vi "Mercury Temperature monitor 2.vi"() -> ()   [LabVIEW 2014]
uses:
  <vilib>/Utility/file.llb/Write To Spreadsheet File (DBL).vi
panel:
  in  "Data Information":string
  out "Needle valve gearing":dbl
  in  "Needle valve gearing":i8
  in  "Needle valve position":dbl(slide) scale=0.0..100.0
  out "Flow set":bool
  out "He-4 flow":dbl
  in  "K pot heater voltage":dbl
  in  "K pot heater":bool
  out "He-3 pot HTR voltage":dbl
  out "Sorb HTR voltage":dbl
  in  "Sorb heater voltage":dbl
  in  "Sorb heater":bool
  out "Sorb Graph":dbl[][](graph)
  in  "seconds to wait":u32=1
  out "General Graph":dbl[][](graph)
  out "He-3 high":dbl
  out "He-3 low":dbl
  out "K pot":dbl
  out "Sorb":dbl
  in  "stop":bool
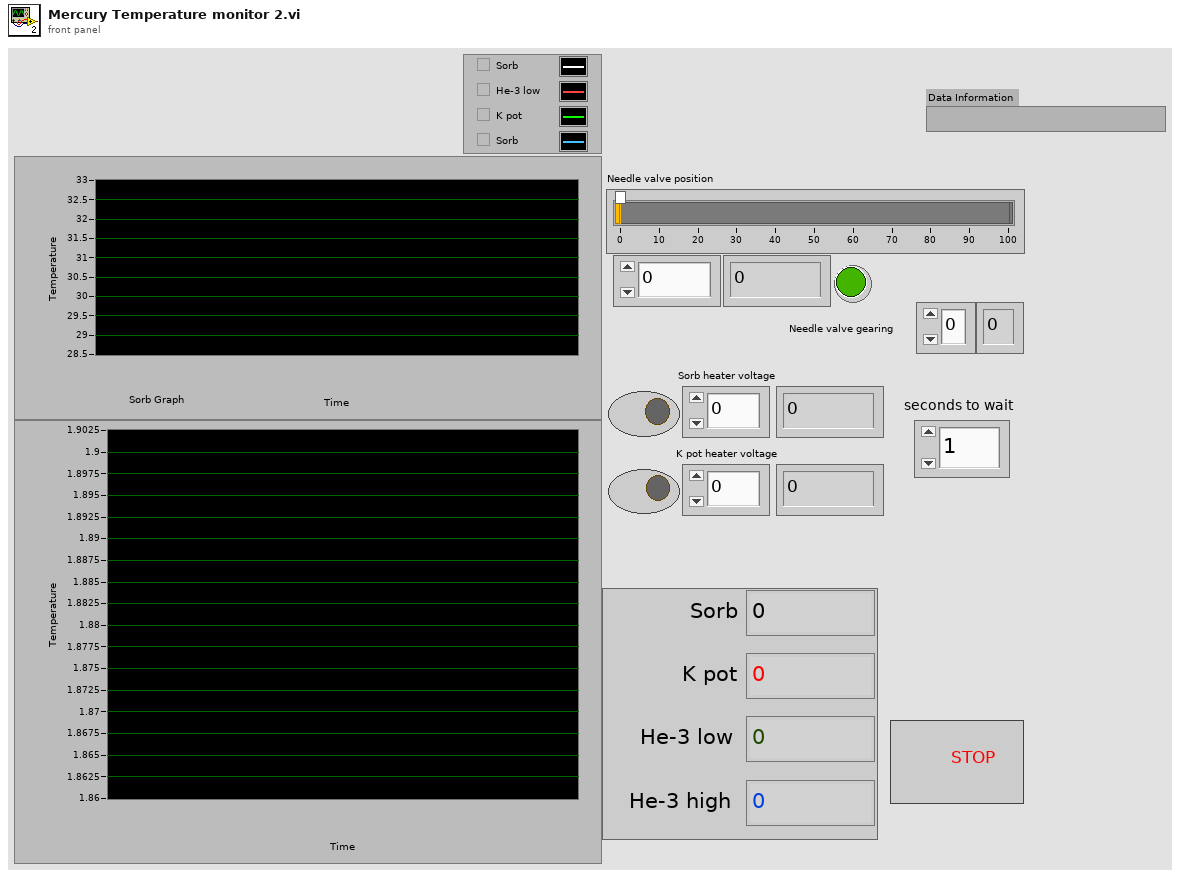
[diagram p1: front panel]
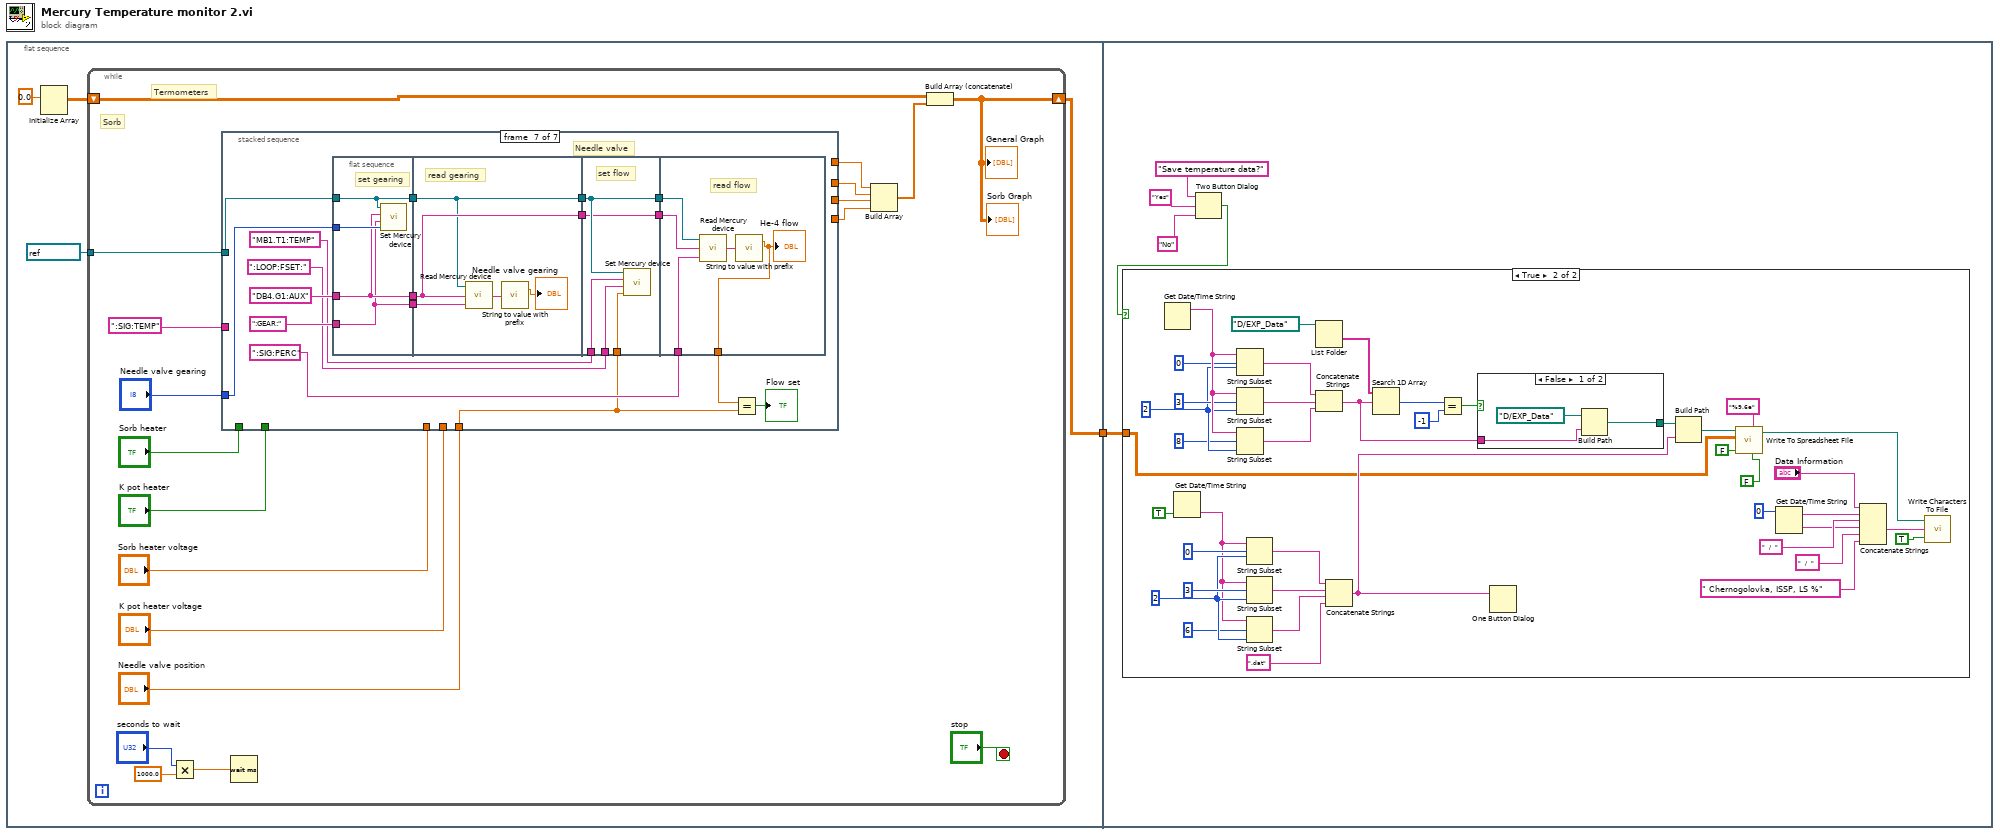
[diagram p0: block diagram]
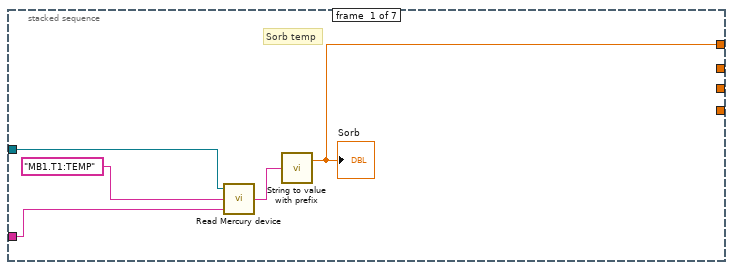
[diagram p2: hidden frame]
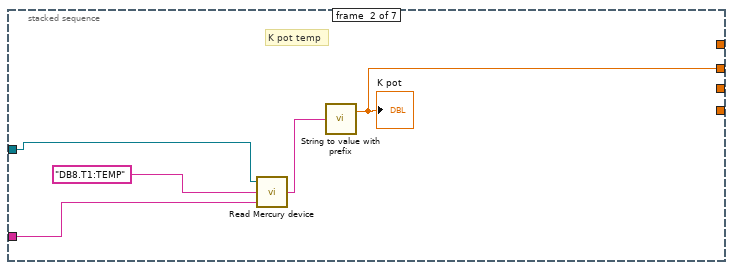
[diagram p3: hidden frame]
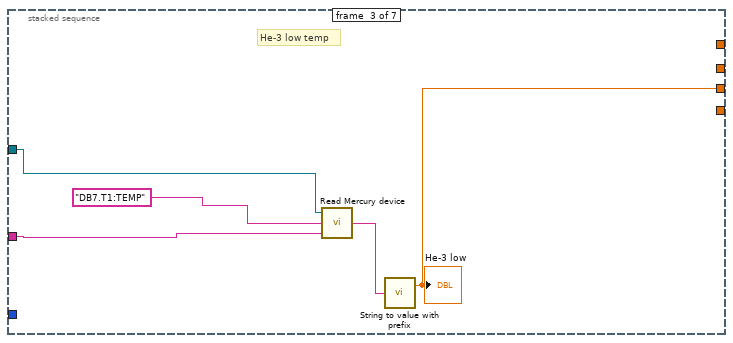
[diagram p4: hidden frame]
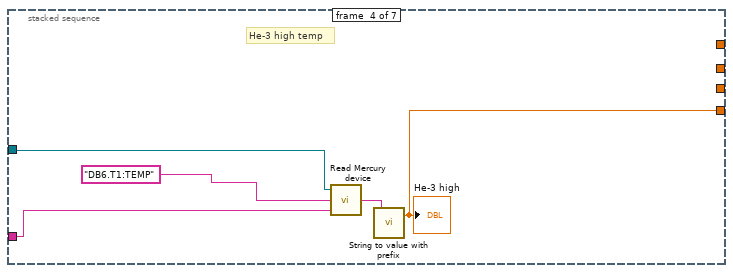
[diagram p5: hidden frame]
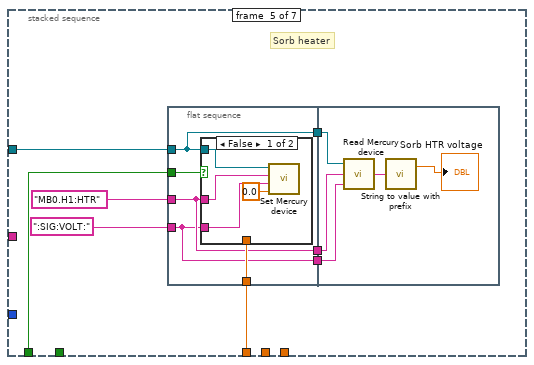
[diagram p6: hidden frame]
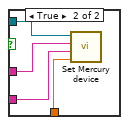
[diagram p7: hidden frame]
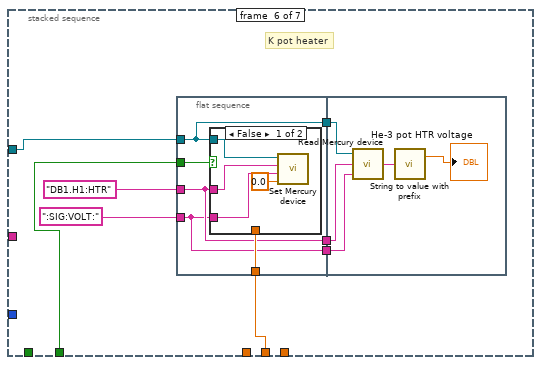
[diagram p8: hidden frame]
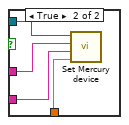
[diagram p9: hidden frame]
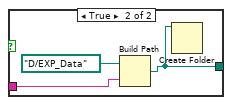
[diagram p11: hidden frame]
diagram:
  n1 = flat-sequence {
    tunnel: [w2] -> w1
    tunnel: w1 -> [w133]
    frame #0 {
      n2 = Initialize Array(0.0 ("element")) -> (w3:dbl[][])  [unwired: 2 in]
      n3 = while {
        shift-right: [w6] -> w2
        shift-left: w3 -> [w7]
        tunnel: refnum<visa-resource-name> "COM4" ("VISA resource name") -> [w23]
        stop <- "stop" stop-if-true
        # "Sorb"
        # "Termometers"
        n4 = Multiply(x="seconds to wait", y=1000.0) -> (x*y=w17:dbl)
        n5 = stacked-sequence {
          tunnel: w23 -> [w29 w33 w39 w43 w48 w73 w112]
          tunnel: ":SIG:TEMP" -> [w28 w34 w38 w42 _ _ _]
          tunnel: [w25 _ _ _ _ _ _] -> w15
          tunnel: [_ w30 _ _ _ _ _] -> w21
          tunnel: [_ _ w35 _ _ _ _] -> w20
          tunnel: [_ _ _ w40 _ _ _] -> w19
          tunnel: "Sorb heater" -> [_ _ _ _ w52 _ _]
          tunnel: "Sorb heater voltage" -> [_ _ _ _ w49 _ _]
          tunnel: "K pot heater" -> [_ _ _ _ _ w72 _]
          tunnel: "K pot heater voltage" -> [_ _ _ _ _ w71 _]
          tunnel: "Needle valve position" -> [_ _ _ _ _ _ w108]
          tunnel: "Needle valve gearing" -> [_ _ _ _ _ _ w105]
          frame #0 {
            # "Sorb temp"
            n6 = call "Read Mercury device.vi"("Additional command"=w28, "Device name"="MB1.T1:TEMP" ("Device Identifier"), "VISA resource name"=w29) -> ("read buffer"=w26:string)
            n7 = call "String to value with prefix.vi"("Incoming string"=w26) -> ("Value"=w25:dbl)  [unwired: 1 out]
            "Sorb" <- w25
          }
          frame #1 {
            # "K pot temp"
            n8 = call "Read Mercury device.vi"("Additional command"=w34, "Device name"="DB8.T1:TEMP" ("Device Identifier"), "VISA resource name"=w33) -> ("read buffer"=w31:string)
            n9 = call "String to value with prefix.vi"("Incoming string"=w31) -> ("Value"=w30:dbl)  [unwired: 1 out]
            "K pot" <- w30
          }
          frame #2 {
            # "He-3 low temp"
            n10 = call "Read Mercury device.vi"("Additional command"=w38, "Device name"="DB7.T1:TEMP" ("Device Identifier"), "VISA resource name"=w39) -> ("read buffer"=w36:string)
            n11 = call "String to value with prefix.vi"("Incoming string"=w36) -> ("Value"=w35:dbl)  [unwired: 1 out]
            "He-3 low" <- w35
          }
          frame #3 {
            # "He-3 high temp"
            n12 = call "Read Mercury device.vi"("Additional command"=w42, "Device name"="DB6.T1:TEMP" ("Device Identifier"), "VISA resource name"=w43) -> ("read buffer"=w41:string)
            n13 = call "String to value with prefix.vi"("Incoming string"=w41) -> ("Value"=w40:dbl)  [unwired: 1 out]
            "He-3 high" <- w40
          }
          frame #4 {
            # "Sorb heater"
            n14 = flat-sequence {
              tunnel: w52 -> [w57]
              tunnel: "MB0.H1:HTR" ("Device Identifier") -> [w54]
              tunnel: ":SIG:VOLT:" ("Device Identifier") -> [w53]
              tunnel: w49 -> [w56]
              tunnel: w48 -> [w55]
              tunnel: [w55] -> w47
              tunnel: [w54] -> w46
              tunnel: [w53] -> w45
              tunnel: w47 -> [w70]
              tunnel: w46 -> [w69]
              tunnel: w45 -> [w68]
              frame #0 {
                n15 = case shown="False" w57 {
                  tunnel: w54 -> [w60 w65]
                  tunnel: w53 -> [w59 w64]
                  tunnel: w56 -> [_ w63]
                  tunnel: w55 -> [w61 w62]
                  frame False {
                    n16 = call "Set Mercury device.vi"("Value"=0.0, "Additional command"=w59, "Device name"=w60, "VISA resource name"=w61) -> ()  [unwired: 1 out]
                  }
                  frame True {
                    n17 = call "Set Mercury device.vi"("Value"=w63, "Additional command"=w64, "Device name"=w65, "VISA resource name"=w62) -> ()  [unwired: 1 out]
                  }
                }
              }
              frame #1 {
                n18 = call "Read Mercury device.vi"("Additional command"=w68, "Device name"=w69, "VISA resource name"=w70) -> ("read buffer"=w67:string)
                n19 = call "String to value with prefix.vi"("Incoming string"=w67) -> ("Value"=→"Sorb HTR voltage":dbl)  [unwired: 1 out]
              }
            }
          }
          frame #5 {
            # "K pot heater"
            n20 = flat-sequence {
              tunnel: w72 -> [w83]
              tunnel: "DB1.H1:HTR" ("Device Identifier") -> [w80]
              tunnel: ":SIG:VOLT:" ("Device Identifier") -> [w79]
              tunnel: w71 -> [w82]
              tunnel: w73 -> [w81]
              tunnel: [w81] -> w78
              tunnel: [w80] -> w77
              tunnel: [w79] -> w76
              tunnel: w78 -> [w96]
              tunnel: w77 -> [w95]
              tunnel: w76 -> [w94]
              frame #0 {
                n21 = case shown="False" w83 {
                  tunnel: w80 -> [w86 w91]
                  tunnel: w79 -> [w85 w90]
                  tunnel: w82 -> [_ w89]
                  tunnel: w81 -> [w87 w88]
                  frame False {
                    n22 = call "Set Mercury device.vi"("Value"=0.0, "Additional command"=w85, "Device name"=w86, "VISA resource name"=w87) -> ()  [unwired: 1 out]
                  }
                  frame True {
                    n23 = call "Set Mercury device.vi"("Value"=w89, "Additional command"=w90, "Device name"=w91, "VISA resource name"=w88) -> ()  [unwired: 1 out]
                  }
                }
              }
              frame #1 {
                n24 = call "Read Mercury device.vi"("Additional command"=w94, "Device name"=w95, "VISA resource name"=w96) -> ("read buffer"=w93:string)
                n25 = call "String to value with prefix.vi"("Incoming string"=w93) -> ("Value"=→"He-3 pot HTR voltage":dbl)  [unwired: 1 out]
              }
            }
          }
          frame #6 {
            # "Needle valve"
            n26 = flat-sequence {
              tunnel: w112 -> [w117]
              tunnel: [w117] -> w104
              tunnel: "DB4.G1:AUX" ("Device Identifier") -> [w115]
              tunnel: ":GEAR:" ("Additional command") -> [w114]
              tunnel: w105 -> [w116]
              tunnel: [w115] -> w100
              tunnel: [w114] -> w97
              tunnel: w104 -> [w119]
              tunnel: [w119] -> w103
              tunnel: w100 -> [w120]
              tunnel: [w120] -> w99
              tunnel: w97 -> [w118]
              tunnel: w108 -> [w127]
              tunnel: [w126] -> w113
              tunnel: w103 -> [w126]
              tunnel: "MB1.T1:TEMP" ("Device Identifier") -> [w125]
              tunnel: ":LOOP:FSET:" ("Device Identifier") -> [w124]
              tunnel: w99 -> [w123]
              tunnel: [w123] -> w98
              tunnel: w113 -> [w132]
              tunnel: ":SIG:PERC" ("Additional command") -> [w130]
              tunnel: [w129] -> w109
              tunnel: w98 -> [w128]
              frame #0 {
                # "set gearing"
                n27 = call "Set Mercury device.vi"("Value"=w116, "Additional command"=w114, "Device name"=w115, "VISA resource name"=w117) -> ()  [unwired: 1 out]
              }
              frame #1 {
                # "read gearing"
                n28 = call "Read Mercury device.vi"("Additional command"=w118, "Device name"=w120, "VISA resource name"=w119) -> ("read buffer"=w122:string)
                n29 = call "String to value with prefix.vi"("Incoming string"=w122) -> ("Value"=→"Needle valve gearing":dbl)  [unwired: 1 out]
              }
              frame #2 {
                # "set flow"
                n30 = call "Set Mercury device.vi"("Value"=w127, "Additional command"=w124, "Device name"=w125, "VISA resource name"=w126) -> ()  [unwired: 1 out]
              }
              frame #3 {
                # "read flow"
                n31 = call "Read Mercury device.vi"("Additional command"=w130, "Device name"=w128, "VISA resource name"=w132) -> ("read buffer"=w131:string)
                n32 = call "String to value with prefix.vi"("Incoming string"=w131) -> ("Value"=w129:dbl)  [unwired: 1 out]
                "He-4 flow" <- w129
              }
            }
            n33 = Equal?(x=w109, y=w108) -> (x = y?=→"Flow set":bool)
          }
        }
        n34 = Wait (ms)(milliseconds to wait=w17) -> ()  [unwired: 1 out]
        n35 = Build Array(w15, w21, w20, w19) -> (w18:dbl[])
        n36 = Build Array (concatenate)(w7, w18) -> (w6:dbl[][])
        "General Graph" <- w6
        "Sorb Graph" <- w6
      }
    }
    frame #1 {
      n37 = Two Button Dialog(message="Save temperature data?", 1:"No" ("F button name (\"Cancel\")"), 2:"Yes" ("T button name (\"OK\")")) -> (T button?=w134:bool)
      n38 = case shown="True" w134 {
        tunnel: w133 -> [_ w139]
        frame False {
        }
        frame True {
          w162 = 2 ("length")
          w174 = 2 ("length")
          n39 = Get Date/Time String() -> (date string=w178:string)  [unwired: 3 in, 1 out]
          n40 = Get Date/Time String(want seconds? (F)=TRUE) -> (time string=w138:string)  [unwired: 2 in, 1 out]
          n41 = String Subset(string=w178, offset (0)=0, length (rest)=w174) -> (substring=w176:string)
          n42 = String Subset(string=w178, offset (0)=3, length (rest)=w174) -> (substring=w172:string)
          n43 = String Subset(string=w178, offset (0)=8, length (rest)=w174) -> (substring=w171:string)
          n44 = String Subset(string=w138, offset (0)=0, length (rest)=w162) -> (substring=w164:string)
          n45 = String Subset(string=w138, offset (0)=3, length (rest)=w162) -> (substring=w160:string)
          n46 = String Subset(string=w138, offset (0)=6, length (rest)=w162) -> (substring=w159:string)
          n47 = List Folder(path=path "D:/EXP_Data") -> (folder names=w140:string[])  [unwired: 3 in, 3 out]
          n48 = Concatenate Strings(w176, w172, w171) -> (w166:string)
          n49 = Concatenate Strings(w164, w160, w159, ".dat" ("string")) -> (w155:string)
          n50 = Search 1D Array(1D array=w140, element=w166) -> (index of element=w169:i32)  [unwired: 1 in]
          n51 = Equal?(x=w169, y=-1) -> (x = y?=w167:bool)
          n52 = case shown="False" w167 {
            tunnel: w166 -> [w180 w184]
            tunnel: [w179 w182] -> w156
            frame False {
              n53 = Build Path(base path=path "D:/EXP_Data", name or relative path=w180) -> (appended path=w179:path)
            }
            frame True {
              n54 = Build Path(base path=path "D:/EXP_Data", name or relative path=w184) -> (appended path=w182:path)
              n55 = Create Folder(path (use dialog)=w182) -> ()  [unwired: 2 in, 3 out]
            }
          }
          n56 = One Button Dialog(message=w155) -> ()  [unwired: 1 in, 1 out]
          n57 = Build Path(base path=w156, name or relative path=w155) -> (appended path=w141:path)
          n58 = call-poly <vilib>:"Write To Spreadsheet File.vi"("transpose? (no:F)"=FALSE, "format (%.3f)"="%9.6e", "append to file? (new file:F)"=FALSE, "2D data"=w139, "file path (dialog if empty)"=w141) -> ("new file path (Not A Path if cancelled)"=w145:path)  [unwired: 3 in]
          n59 = Get Date/Time String(date format (0)=0) -> (date string=w150:string, time string=w151:string)  [unwired: 2 in]
          n60 = Concatenate Strings("Data Information", w150, "  /  " ("date string"), w151, "  /  " ("date string"), " Chernogolovka, ISSP, LS %" ("date string")) -> (w148:string)
          n61 = call <vilib>:"Write Characters To File.vi"("append to file? (new file:F)"=TRUE, "character string"=w148, "file path (dialog if empty)"=w145) -> ()  [unwired: 2 in, 1 out]
        }
      }
    }
  }
